vi "MoveRotaryArm.vi"(8 "error in (no error)":errorcluster caption="Fehler (Eingang, kein Fehler)", 9 "Speed":i16=50, 10 "Rotary Arm":dbl, 11 "Moveo Eingang":refnum<class "Moveo.lvclass">) -> (0 "error out":errorcluster caption="Fehler (Ausgang)", 3 "Moveo Ausgang":refnum<class "Moveo.lvclass">)   [LabVIEW 2019, in "Moveo.lvclass"]
uses:
  Moveo.lvclass
  Moveo.lvclass/Moveo.ctl
  MoveoSerialClass/MoveoSerial.lvclass
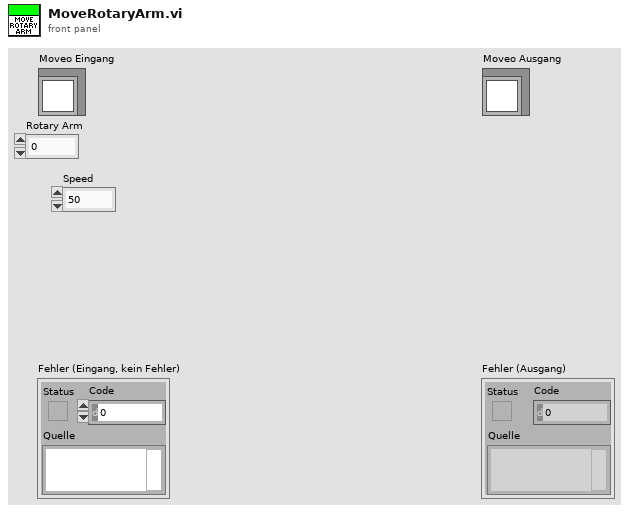
[diagram p1: front panel]
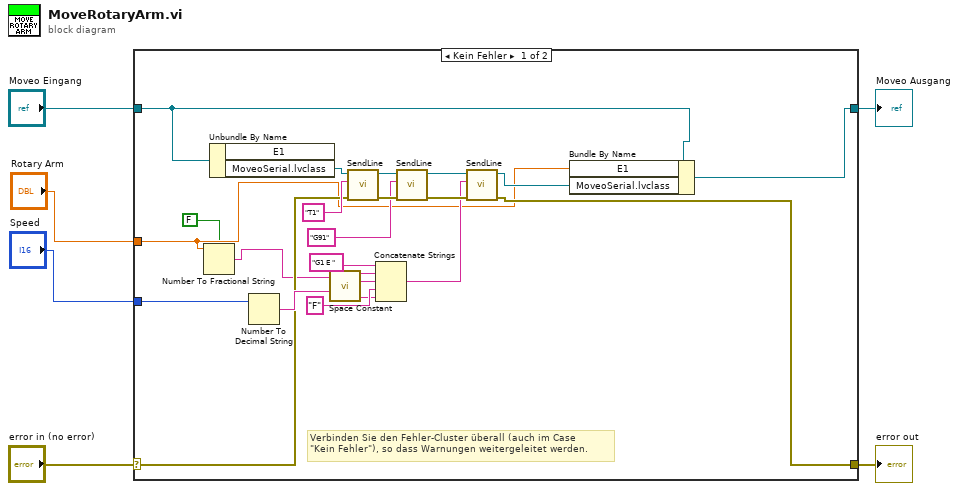
[diagram p0: block diagram]
diagram:
  n1 = case shown="Kein Fehler" "error in (no error)" {
    selector: "error in (no error)" -> [w11 w29]
    tunnel: [w10 w29] -> w5
    tunnel: [w13 w28] -> w3
    tunnel: "Moveo Eingang" -> [w14 w28]
    tunnel: "Speed" -> [w12 _]
    tunnel: "Rotary Arm" -> [w8 _]
    frame No Error {
      # "Verbinden Sie den Fehler-Cluster überall (auch im Case\n\"Kein Fehler\"), so dass Warnungen weitergeleitet werden."
      n2 = Number To Fractional String(use system decimal point (T)=FALSE ("Systemdezimalzeichen verwenden (T)"), number=w8) -> (F-format string=w9:string)  [unwired: 2 in]
      n3 = Unbundle By Name(w14) -> ("MoveoSerial.lvclass"=w27:refnum<class "MoveoSerial.lvclass">)  [unwired: 1 out]
      n4 = Number To Decimal String(number=w12) -> (decimal integer string=w19:string)  [unwired: 1 in]
      n5 = call <vilib>:"Space Constant.vi"() -> ("String"=w21:string)
      n6 = call-dynamic "SendLine.vi"("error in (no error)"=w11, "SendString"="T1", "MoveoSerial Eingang"=w27) -> ("error out"=w25:errorcluster, "MoveoSerial Ausgang"=w24:refnum<class "MoveoSerial.lvclass">)  [unwired: 7 in]
      n7 = Concatenate Strings("G1 E ", w9, w21, "F", w19) -> (w16:string)
      n8 = call-dynamic "SendLine.vi"("error in (no error)"=w25, "SendString"="G91", "MoveoSerial Eingang"=w24) -> ("error out"=w17:errorcluster, "MoveoSerial Ausgang"=w18:refnum<class "MoveoSerial.lvclass">)  [unwired: 7 in]
      n9 = call-dynamic "SendLine.vi"("error in (no error)"=w17, "SendString"=w16, "MoveoSerial Eingang"=w18) -> ("error out"=w10:errorcluster, "MoveoSerial Ausgang"=w15:refnum<class "MoveoSerial.lvclass">)  [unwired: 7 in]
      n10 = Bundle By Name(cluster=w14, "E1"=w8, "MoveoSerial.lvclass"=w15) -> (w13:refnum<class "Moveo.lvclass">)
    }
    frame Error {
    }
  }
  "error out" <- w5
  "Moveo Ausgang" <- w3
